vi "Delete Source Files Missing From Install.vi"(8 "Error In":errorcluster, 10 "Source Files":path[](array[path]), 11 "Configuration":T1) -> (0 "Error Out":errorcluster, 2 "Deleted From Souce":path[](array[path]), 3 "Configuration":T1)   [LabVIEW 2011, in "LVH-Toolbox.lvlib" / "LVH-Build-Tools.lvlib"]
uses:
  LVH-Build-Tools.lvlib
  Type Defs/Configuration.ctl
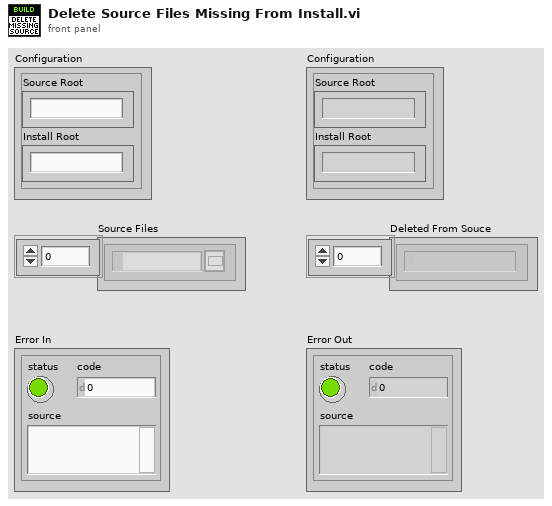
[diagram p1: front panel]
types:
  T1 = typedef "LVH-Toolbox.lvlib/LVH-Build-Tools.lvlib/Configuration.ctl" = cluster{"Source Root":string, "Install Root":string, "Components":string[], "Ignore":string[]}
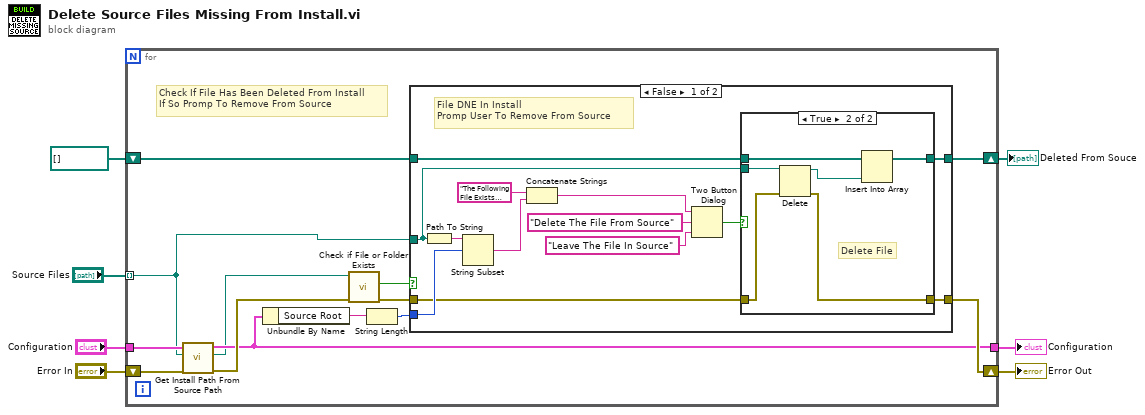
[diagram p0: block diagram]
diagram:
  n1 = for {
    tunnel: "Configuration" -> [w12]
    tunnel: "Source Files" -> [w8] mode=indexing
    shift-right: [w15] -> w7
    shift-left: "Error In" -> [w20]
    tunnel: [w11] -> w1
    shift-right: [w13] -> w6
    shift-left: path[] [] ("Array in") -> [w14]
    # "Check If File Has Been Deleted From Install \nIf So Promp To Remove From Source"
    n2 = call "Get Install Path From Source Path.vi"("Error In"=w20, "Source File Path"=w8, "Configuration"=w12) -> ("Error Out"=w19:errorcluster, "Install File Path"=w9:path, "Configuration"=w11:T1)  [unwired: 5 in, 1 out]
    n3 = Unbundle By Name(w11) -> ("Source Root"=w10:string)
    n4 = call <vilib>:"Check if File or Folder Exists.vi"("error in (no error)"=w19, "path"=w9) -> ("error out"=w17:errorcluster, "file or folder exists?"=w18:bool)  [unwired: 7 in, 1 out]
    n5 = String Length(string=w10) -> (length=w16:i32)
    n6 = case shown="False" w18 {
      tunnel: w8 -> [w25 _]
      tunnel: w17 -> [w24 w43]
      tunnel: w16 -> [w31 _]
      tunnel: [w23 w43] -> w15
      tunnel: w14 -> [w22 w42]
      tunnel: [w21 w42] -> w13
      frame False {
        # "File DNE In Install\nPromp User To Remove From Source"
        n7 = Path To String(path=w25) -> (string=w32:string)
        n8 = String Subset(string=w32, offset (0)=w31) -> (substring=w30:string)  [unwired: 1 in]
        n9 = Concatenate Strings("The Following File Exists Under The Source Directory But Not The Install Directory.\n\n", w30) -> (w29:string)
        n10 = Two Button Dialog(message=w29, 1:"Leave The File In Source" ("F button name (\"Cancel\")"), 2:"Delete The File From Source" ("T button name (\"OK\")")) -> (T button?=w26:bool)
        n11 = case shown="True" w26 {
          tunnel: w25 -> [_ w41]
          tunnel: w24 -> [w35 w40]
          tunnel: [w35 w39] -> w23
          tunnel: w22 -> [w34 w38]
          tunnel: [w34 w36] -> w21
          frame False {
            # "Leave File"
          }
          frame True {
            # "Delete File"
            n12 = Delete(path (use dialog)=w41, error in=w40) -> (deleted path=w37:path, error out=w39:errorcluster)  [unwired: 3 in, 1 out]
            n13 = Insert Into Array(array=w38, new element=w37) -> (w36:path[])  [unwired: 1 in]
          }
        }
      }
      frame True {
        # "File Exists In Source And Install.  Move On."
      }
    }
  }
  "Error Out" <- w7
  "Deleted From Souce" <- w6
  "Configuration" <- w1
